vi "bode_ph.vi"() -> ()   [LabVIEW 2014]
doc: "Bode plot\nAcquisisce la risposta di un circuito utilizzando il generatore interno\nGenera il grafico della risposta in funzione della frequenza\nFM & ADL 09/2009, 10/2012, 10/2013 versione per 8.6 \nModifcato con set di DMA e Interrupts FM 10/2013\n9/2015 vers. LV2014"
uses:
  <vilib>/DAQmx/write.llb/DAQmx Write (Analog 1D DBL 1Chan NSamp).vi
  <vilib>/DAQmx/read.llb/DAQmx Read (Analog 1D Wfm NChan NSamp).vi
  <vilib>/DAQmx/create/channels.llb/DAQmx Create Channel (AO-Voltage-Basic).vi
  <vilib>/DAQmx/create/channels.llb/DAQmx Create Channel (AI-Voltage-Basic).vi
  <vilib>/DAQmx/configure/timing.llb/DAQmx Timing (Sample Clock).vi
  <vilib>/DAQmx/miscellaneous.llb/DAQmx Fill In Error Info.vi
  <vilib>/measure/matone.llb/Extract Single Tone Information 1 Chan.vi
  <vilib>/Utility/file.llb/Write To Spreadsheet File (DBL).vi
  <vilib>/measure/NI_MABase.lvlib
  <vilib>/measure/NI_MAPro.lvlib
  <resource>/objmgr/daqmx.rc
panel:
  in  "Fondo Scala":dbl(ring)=5.0 items=["10"=10.0, "5"=5.0, "0.5"=0.5, "0.05"=0.05]
  out "N. misura":i32=20
  in  "SALVA I DATI SU FILE":bool=TRUE caption="ON\nOFF"
  out "Fase":cluster{dbl[], dbl[]}(graph)={[5.0, 6.147467068473125, 7.558270271592312, 9.29284351784663, 11.42548989968722, 14.047564579899898, 17.271388129436826, 21.23505795050611, 26.10836388957094, 32.10006144457005, 39.46681412529165, 48.52418802655607, 59.66016958353027, 73.35178556285486, 90.18553723227052, 110.882524037588, 136.32933299805035, 167.61601701448424, 206.08278894903452, 253.37743168865742, 311.52588344006404, 383.0190218849582, 470.91936472731345, 578.9922573134888, 711.867166947118, 875.2359931869336, 1076.0968890518084, 1323.054037586474, 1626.6862251746509, 2000.0000000000045], [-2.511428467979215, -3.2956057199072006, -7.538567169946305, -10.113388336699302, -10.892831534570234, -13.380062579809533, -10.774958061787402, -13.590987224260658, -21.65618380795769, -25.567045102139673, -29.374990352035297, -30.80584091335669, -40.39456715017832, -46.922681187413104, -49.46128006672848, -55.656601427298085, -62.68913088564615, -64.84436978845952, -67.56276682724092, -74.50767078379593, -76.96614211460007, -77.43816453034884, -79.04548854172731, -83.2980148193289, -80.94888607866157, -84.03334246814163, -78.13471017673413, -78.78110200061434, -92.0554038069169, -84.81527118746277]}
  out "GAIN":cluster{dbl[], dbl[]}(graph)={[5.0, 6.147467068473125, 7.558270271592312, 9.29284351784663, 11.42548989968722, 14.047564579899898, 17.271388129436826, 21.23505795050611, 26.10836388957094, 32.10006144457005, 39.46681412529165, 48.52418802655607, 59.66016958353027, 73.35178556285486, 90.18553723227052, 110.882524037588, 136.32933299805035, 167.61601701448424, 206.08278894903452, 253.37743168865742, 311.52588344006404, 383.0190218849582, 470.91936472731345, 578.9922573134888, 711.867166947118, 875.2359931869336, 1076.0968890518084, 1323.054037586474, 1626.6862251746509, 2000.0000000000045], [0.997344434549249, 0.9962213082665805, 0.9941210435643523, 0.9922479926095603, 0.9878479615556824, 0.9824573247202957, 0.9738931698701306, 0.9613958789343343, 0.9430943055783031, 0.9186590086551807, 0.88260450854282, 0.8371109796491035, 0.7795638387175756, 0.7122020936433959, 0.6364315890190533, 0.5575733199071561, 0.48003430290297966, 0.4070800618335603, 0.3414788103570544, 0.28392605144903055, 0.23469423754251195, 0.19299749424063478, 0.15862845124464225, 0.1302776763618104, 0.10670713632692706, 0.08756567054703944, 0.07027549073207927, 0.057247542713008, 0.0468367874762694, 0.03824708830461569]}
  out "Vin (bianco) Vout (giallo)":waveform(dbl)[](graph)=[{"t0"=timestamp(3463116182.984375 s since 1904-01-01), "dt"=1.9999999999999998e-05, "Y"=[-0.40354768966159216, -0.3176421394330232, -0.2118748908641203, -0.09250948886795704, 0.032113552093432515, 0.1550167936225486, 0.26847628237502535, 0.3652222773509948, 0.43879623760444986, 0.4845894271489925, 0.5005894831758473, 0.4845894271489925, 0.43879623760444986, 0.3652222773509948, 0.26847628237502535, 0.15478961539836963, 0.03198373631517646, -0.09293138951490015, -0.21213452196228907, -0.31796667853872895, -0.40370995941588605, -0.4641067976603833, -0.49532754826133535, -0.4953600022764232, -0.4641067976603833, -0.4040669528769932, -0.31799913244936345, -0.21232924528602865, -0.09289893561902575, 0.031821466592759425, 0.15478961539836963, 0.268151740898926, 0.36509246025984043, 0.4383418762293826, 0.4846218816097759, 0.5003947562443536, 0.4846867905315109, 0.43860151129959596, 0.3649626431694226, 0.2683140116365024, 0.15482206943031035, 0.03172410475952403, -0.09302875120247918, -0.21216697584957225, -0.31803158636000955, -0.40374241336680144, -0.4640743436696399, -0.4953924562915376, -0.49532754826133535, -0.4641717056419421, -0.4039046831216613, -0.31803158636000955, -0.21229679139873198, -0.09293138951490015, 0.031886374481672516, 0.15462734523909027, 0.2682815574889114, 0.3648003718074358, 0.43853660253172927, 0.4846867905315109, 0.5002973927793823, 0.48471924499246266, 0.43853660253172927, 0.3649626431694226, 0.26834646578413124, 0.1546597992708896, 0.031756558703917935, -0.09280157393135828, -0.21203716030045566, -0.3178693168068953, -0.40374241336680144, -0.4640094356882249, -0.4951977322012501, -0.49532754826133535, -0.46394452770690575, -0.40370995941588605, -0.3180964941813367, -0.21223188362414672, -0.09302875120247918, 0.03185392053720702, 0.15452998314386185, 0.268216649193843, 0.3648977346244899, 0.4386339656836077, 0.4844920637669791, 0.5004596652212883, 0.4846867905315109, 0.4385690569156365, 0.3649626431694226, 0.26834646578413124, 0.15482206943031035, 0.03195128237065724, -0.09289893561902575, -0.2121020680750086, -0.31803158636000955, -0.4038722291706516, -0.4641067976603833, -0.4952301862162315, -0.4953924562915376, -0.4640094356882249, -0.4039695910237374, -0.3179342246281061, -0.2121020680750086, -0.09296384341076719, 0.031918828426155926, 0.15482206943031035, 0.268443828227245, 0.36518982307813713, 0.43866642006767165, 0.48471924499246266, 0.5004596652212883, 0.48471924499246266, 0.43869887445178785, 0.36518982307813713, 0.2682815574889114, 0.1548869774942766, 0.031886374481672516, -0.09280157393135828, -0.21203716030045566, -0.3178368628963073, -0.4038073212686888, -0.46391207371628207, -0.4953924562915376, -0.4951977322012501, -0.4641392516511507], "attributes"=variant("NI_ChannelName"=variant(string "Dev1/ai0"), "NI_UnitDescription"=variant(string "Volts"))}, {"t0"=timestamp(3463116182.984385 s since 1904-01-01), "dt"=1.9999999999999998e-05, "Y"=[-0.011212449060798765, -0.014522749144446944, -0.0166647079443697, -0.0177032334014217, -0.017670779481101948, -0.01627526089433491, -0.014003486395925527, -0.010530916672304998, -0.006246998656095383, -0.001800810747352719, 0.003067278528288692, 0.007902914220070749, 0.011992109777829095, 0.015562042618044544, 0.018255719347841527, 0.01994332410473799, 0.020332771362804047, 0.01971614653865677, 0.018060995724968443, 0.015140141453851102, 0.011343031100809003, 0.006961750199018043, 0.00222347636249437, -0.0026446128537431536, -0.007188162484401767, -0.011050179445062374, -0.01429557169241011, -0.01676206970656755, -0.01780059516229866, -0.017476055958895155, -0.016210353052468814, -0.013743855020318461, -0.010336193131576134, -0.006311906506719184, -0.0016060871828953507, 0.0029374628097945813, 0.007675736696527374, 0.011764932240134893, 0.015432226874918577, 0.01812590359919249, 0.020040685919026205, 0.020430133177701308, 0.019813508352590256, 0.01786627210269795, 0.015042779647125564, 0.01118076143256555, 0.006799480541560849, 0.0019638449289622025, -0.0026770667807093336, -0.007415339958356825, -0.01124490298390323, -0.014555203066110517, -0.016599800102835436, -0.017897956923052214, -0.017476055958895155, -0.01634016873614565, -0.01384121678627644, -0.010758094135836926, -0.00637681435728426, -0.0019630803839862975, 0.0033593638958058698, 0.007416105242000887, 0.01186229404190654, 0.015367319003454703, 0.018190811473483507, 0.01987841622863034, 0.02062485680795324, 0.019521422911245437, 0.017768910291788485, 0.01481560209867611, 0.011050945698261642, 0.006572303021783793, 0.0018664831416414804, -0.0029691521227308277, -0.007480247807926938, -0.011472080445235226, -0.014522749144446944, -0.0166647079443697, -0.017768141242020054, -0.0177032334014217, -0.016210353052468814, -0.014068394239686921, -0.010628278442476005, -0.006539083983440174, -0.002125350020243671, 0.002710285303025065, 0.007286289515117891, 0.011797386174042565, 0.015399772939178383, 0.018158357536329627, 0.019845962290601853, 0.020397679239385288, 0.019456515035576584, 0.017639094544143183, 0.014718240292444796, 0.010856222097290128, 0.006539849090450168, 0.0018015752835045273, -0.002871790342191765, -0.007350432108728361, -0.010952817675449186, -0.014522749144446944, -0.01676206970656755, -0.017897956923052214, -0.017962864763486065, -0.01653489226124592, -0.01423066384884499, -0.010952817675449186, -0.007025892859709993, -0.0022876196561251814, 0.002612923514641253, 0.00731874344681489, 0.01173247830624343, 0.015432226874918577, 0.01796363391375791, 0.01958633078698174, 0.020040685919026205, 0.01948896897340258, 0.017541732733584593, 0.014555970615721696, 0.010953583897703262, 0.006474941227830212, 0.0017366674254290385, -0.002871790342191765, -0.0073828860335498885], "attributes"=variant("NI_ChannelName"=variant(string "Dev1/ai1"), "NI_UnitDescription"=variant(string "Volts"))}]
  out "f_attuale":dbl=2000.0000000000045
  out "Ncamp/periodo":dbl=25.0
  in  "Nperiodi":dbl=5.0
  in  "Numero misure":i16=30
  in  "Freqmax":dbl=2000.0 min=0.0 max=100000.0
  in  "Freqmin":dbl=5.0 min=0.0 max=100000.0
  # "1) Scegliere la frequenza iniziale e finale (<8 kHz) e il numero di misure.\n2) Scegliere quanti periodi della sinusoide si prendono e quanti campioni si generano per ogni periodo; per le frequenze alte ridurre il NCamp/periodo: il prodotto Freqmax * Ncamp non deve superare  ~ 60000.\n3) Premere la freccia bianca di avvio."
  # "Foma d'onda generata Vin(t)"
  # "NO\nSI"
  # "Fase"
  # "I Collegamenti"
  # "Collegare il CB 22 (Analog Output 0) all'ingresso. \nI due canali di misura (riferiti a terra) sono il CB68 (Vin) e CB33 (Vout).\nLa terra del circuito DEVE essere in comune alla terra della scheda (CB29)."
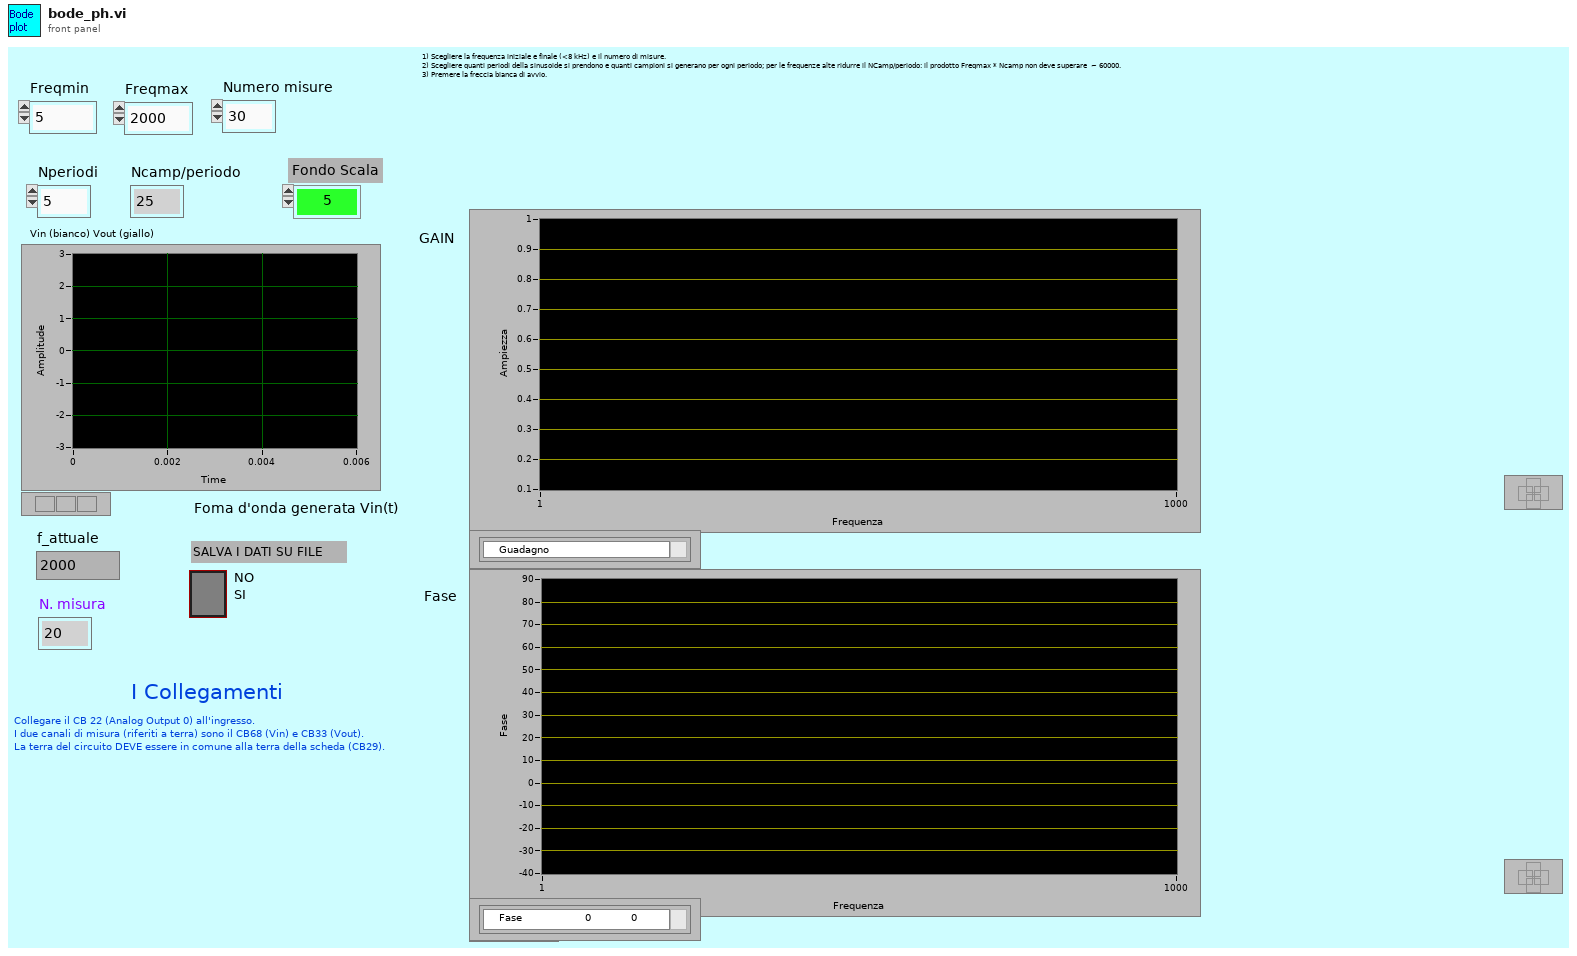
[diagram p1: front panel]
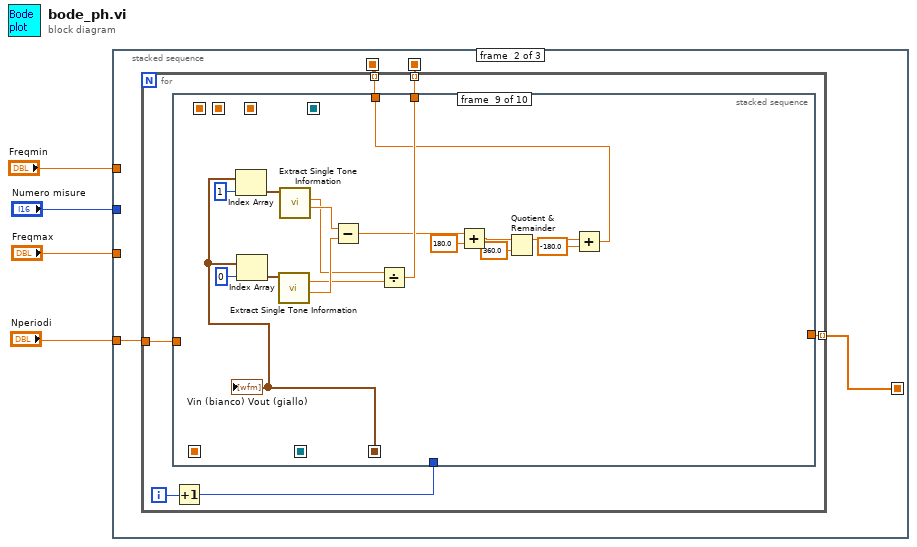
[diagram p0: block diagram]
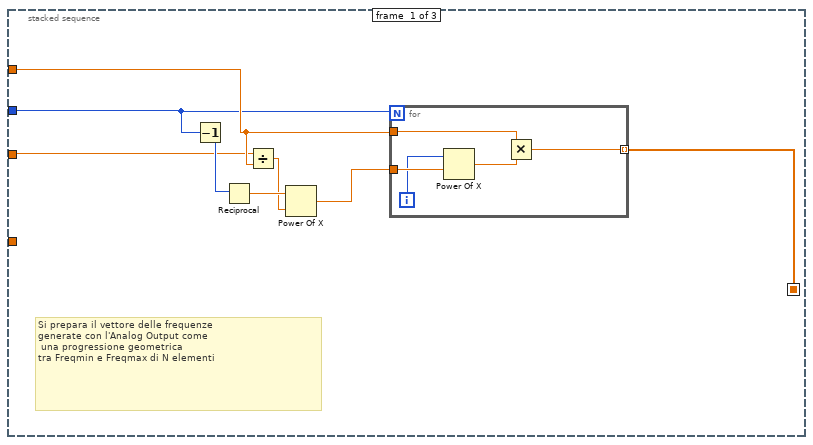
[diagram p2: hidden frame]
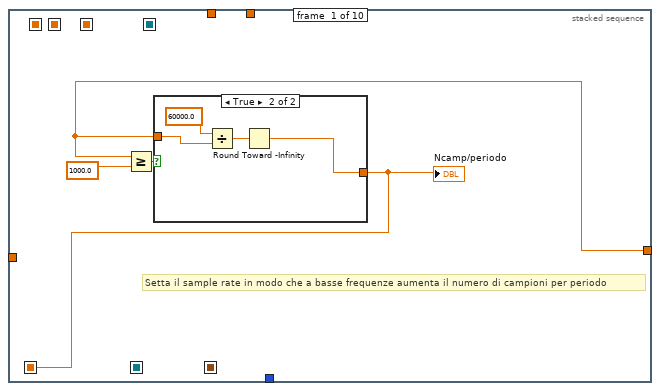
[diagram p3: hidden frame]
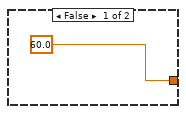
[diagram p4: hidden frame]
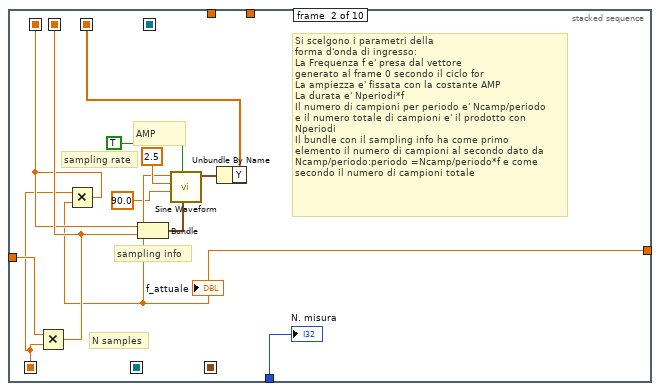
[diagram p5: hidden frame]
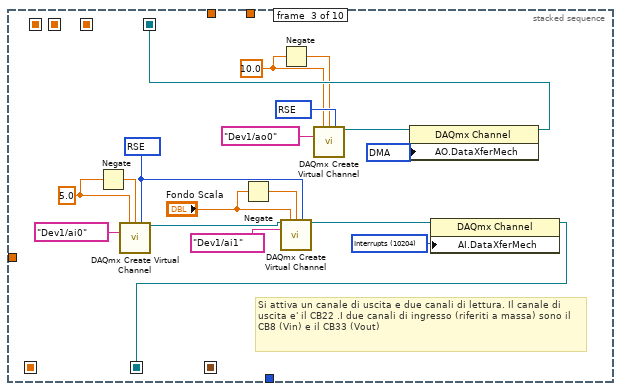
[diagram p6: hidden frame]
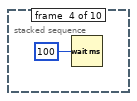
[diagram p7: hidden frame]
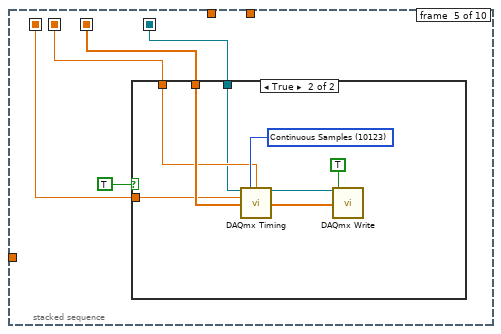
[diagram p8: hidden frame]
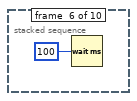
[diagram p10: hidden frame]
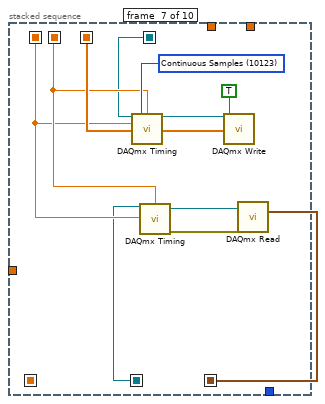
[diagram p11: hidden frame]
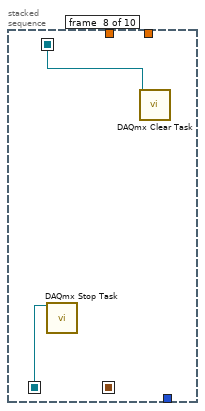
[diagram p12: hidden frame]
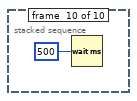
[diagram p13: hidden frame]
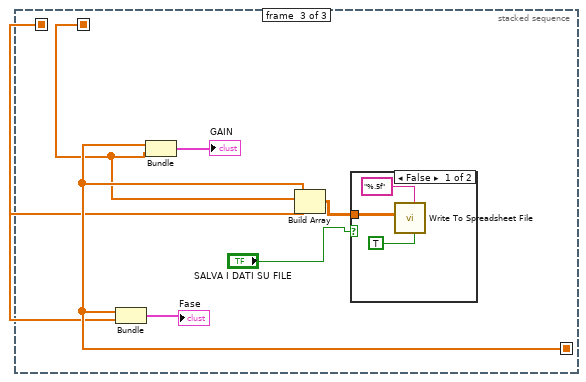
[diagram p14: hidden frame]
diagram:
  n1 = stacked-sequence {
    seq-local: [w5 _ _] -> [_ w21 w116]
    seq-local: [_ w19 _] -> [_ _ w115]
    seq-local: [_ w18 _] -> [_ _ w114]
    tunnel: "Freqmin" -> [w8 _ _]
    tunnel: "Numero misure" -> [w7 _ _]
    tunnel: "Freqmax" -> [w6 _ _]
    tunnel: "Nperiodi" -> [_ w20 _]
    frame #0 {
      # "Si prepara il vettore delle frequenze\ngenerate con l'Analog Output come\n una progressione geometrica\ntra Freqmin e Freqmax di N elementi"
      n2 = Decrement(x=w7) -> (x-1=w12:i16)
      n3 = Reciprocal(x=w12) -> (1/x=w11:dbl)
      n4 = Divide(x=w6, y=w8) -> (x/y=w10:dbl)
      n5 = Power Of X(1:w10, 2:w11) -> (0:w9:dbl)
      n6 = for {
        N: w7 -> [_]
        tunnel: w9 -> [w17]
        tunnel: w8 -> [w15]
        tunnel: [w13] -> w5 mode=indexing
        i -> [w16]
        n7 = Power Of X(1:w17, 2:w16) -> (0:w14:dbl)
        n8 = Multiply(x=w15, y=w14) -> (x*y=w13:dbl)
      }
    }
    frame #1 {
      n9 = for {
        tunnel: w21 -> [w24] mode=indexing
        tunnel: w20 -> [w27]
        tunnel: [w26] -> w19 mode=indexing
        tunnel: [w25] -> w18 mode=indexing
        i -> [w23]
        n10 = Increment(x=w23) -> (x+1=w22:i32)
        n11 = stacked-sequence {
          seq-local: [_ w46 _ _ _ _ _ _ _ _] -> [_ _ _ _ w72 _ w86 _ _ _]
          seq-local: [_ w43 _ _ _ _ _ _ _ _] -> [_ _ _ _ w71 _ w84 _ _ _]
          seq-local: [_ w42 _ _ _ _ _ _ _ _] -> [_ _ _ _ w70 _ w83 _ _ _]
          seq-local: [_ _ _ _ _ _ w87 _ _ _] -> [_ _ _ _ _ _ _ _ w108 _]
          seq-local: [w28 _ _ _ _ _ _ _ _ _] -> [_ w38 _ _ _ _ _ _ _ _]
          seq-local: [_ _ w61 _ _ _ _ _ _ _] -> [_ _ _ _ w69 _ w82 w92 _ _]
          seq-local: [_ _ w59 _ _ _ _ _ _ _] -> [_ _ _ _ _ _ w81 w93 _ _]
          tunnel: w24 -> [w29 w41 _ _ _ _ _ _ _ _]
          tunnel: w27 -> [_ w44 _ _ _ _ _ _ _ _]
          tunnel: [_ _ _ _ _ _ _ _ w104 _] -> w26
          tunnel: [_ _ _ _ _ _ _ _ w94 _] -> w25
          tunnel: w22 -> [_ w37 _ _ _ _ _ _ _ _]
          frame #0 {
            # "Setta il sample rate in modo che a basse frequenze aumenta il numero di campioni per periodo"
            n12 = Greater Or Equal?(x=w29, y=1000.0) -> (x >= y?=w30:bool)
            n13 = case shown="True" w30 {
              tunnel: [60.0 w33] -> w28
              tunnel: w29 -> [_ w36]
              frame False {
              }
              frame True {
                n14 = Divide(x=60000.0, y=w36) -> (x/y=w34:dbl)
                n15 = Round Toward -Infinity(1:w34) -> (0:w33:dbl)
              }
            }
            "Ncamp/periodo" <- w28
          }
          frame #1 {
            # "Si scelgono i parametri della\nforma d'onda di ingresso:\nLa Frequenza f e' presa dal vettore \ngenerato al frame 0 secondo il ciclo for\nLa ampiezza e' fissata con la costante AMP\nLa durata e' Nperiodi*f\nIl numero di campioni per periodo e' Ncamp/periodo\ne il numero totale di campioni e' il prodotto con \nNperiodi\nIl bundle con il sampling info ha come primo\nelemento il numero di campioni al secondo dato da \nNcamp/periodo:periodo =Ncamp/periodo*f e come\nsecondo il numero di campioni totale"
            # "sampling rate"
            # "N samples"
            # "AMP"
            # "sampling info"
            n16 = Multiply(x=w44, y=w38) -> (x*y=w43:dbl)
            n17 = Multiply(x=w38, y=w41) -> (x*y=w42:dbl)
            n18 = Bundle(w42, w43) -> (w45:cluster{dbl, dbl})  [unwired: 1 out]
            n19 = call <vilib>:"Sine Waveform.vi"("sampling info"=w45, "reset signal"=TRUE, "phase"=90.0, "amplitude"=2.5, "frequency"=w41) -> ("signal out"=w47:waveform(dbl))  [unwired: 2 in, 4 out]
            n20 = Unbundle By Name(w47) -> ("Y"=w46:dbl[])
            "f_attuale" <- w41
            "N. misura" <- w37
          }
          frame #2 {
            w60 = 10204 items=["DMA"=10054, "Interrupts"=10204, "Programmed I/O"=10264, "USB Bulk"=12590] ("AO.DataXferMech")
            w63 = 10054 items=["DMA"=10054, "Interrupts"=10204, "Programmed I/O"=10264, "USB Bulk"=12590] ("AO.DataXferMech")
            w58 = 5.0 ("maximum value")
            w52 = 10083 items=["default"=-1, "RSE"=10083, "NRSE"=10078, "Differential"=10106, "Pseudodifferential"=12529] ("input terminal configuration")
            w56 = 10.0 ("maximum value")
            w65 = 10083 items=["Default"=-1, "RSE"=10083, "Differential"=10106, "Pseudodifferential"=12529] ("output terminal configuration")
            # "Si attiva un canale di uscita e due canali di lettura. Il canale di uscita e' il CB22 .I due canali di ingresso (riferiti a massa) sono il CB8 (Vin) e il CB33 (Vout)"
            n21 = Negate(x=w58) -> (-x=w57:dbl)
            n22 = call-poly <vilib>:"DAQmx Create Virtual Channel.vi"("maximum value"=w58, "minimum value"=w57, "input terminal configuration"=w52, "physical channels"=tag "Dev1/ai0") -> ("task out"=w53:refnum<k21>)  [unwired: 5 in, 6 out]
            n23 = Negate(x="Fondo Scala") -> (-x=w51:dbl)
            n24 = Negate(x=w56) -> (-x=w55:dbl)
            n25 = call-poly <vilib>:"DAQmx Create Virtual Channel.vi"("task in"=w53, "maximum value"="Fondo Scala", "minimum value"=w51, "input terminal configuration"=w52, "physical channels"=tag "Dev1/ai1") -> ("task out"=w49:refnum<k21>)  [unwired: 4 in, 6 out]
            n26 = call-poly <vilib>:"DAQmx Create Virtual Channel.vi"("maximum value"=w56, "minimum value"=w55, "output terminal configuration"=w65, "physical channels"=tag "Dev1/ao0") -> ("task out"=w62:refnum<k21>)  [unwired: 5 in, 6 out]
            n27 = property class="DAQmx Channel"(reference=w62, "AO.DataXferMech"=w63) -> (reference out=w61:refnum<k21>)  [unwired: 1 in, 1 out]
            n28 = property class="DAQmx Channel"(reference=w49, "AI.DataXferMech"=w60) -> (reference out=w59:refnum<k21>)  [unwired: 1 in, 1 out]
          }
          frame #3 {
            n29 = Wait (ms)(milliseconds to wait=u32 100 ("millisecond multiple")) -> ()  [unwired: 1 out]
          }
          frame #4 {
            n30 = case shown="True" TRUE {
              tunnel: w72 -> [_ w77]
              tunnel: w71 -> [_ w75]
              tunnel: w70 -> [_ w74]
              tunnel: w69 -> [_ w73]
              frame False {
              }
              frame True {
                w76 = 10123 items=["Finite Samples"=10178, "Continuous Samples"=10123, "Hardware Timed Single Point"=12522] ("sample mode")
                n31 = call-poly <vilib>:"DAQmx Timing.vi"("task/channels in"=w73, "sample mode"=w76, "samples per channel"=w75, "rate"=w74) -> ("task out"=w78:refnum<k21>)  [unwired: 3 in, 8 out]
                n32 = call-poly <vilib>:"DAQmx Write.vi"("task/channels in"=w78, "auto start"=TRUE, "data"=w77) -> ()  [unwired: 1 in, 12 out]
              }
            }
          }
          frame #5 {
            n33 = Wait (ms)(milliseconds to wait=u32 100 ("millisecond multiple")) -> ()  [unwired: 1 out]
          }
          frame #6 {
            w85 = 10123 items=["Finite Samples"=10178, "Continuous Samples"=10123, "Hardware Timed Single Point"=12522] ("sample mode")
            n34 = call-poly <vilib>:"DAQmx Timing.vi"("task/channels in"=w82, "sample mode"=w85, "samples per channel"=w84, "rate"=w83) -> ("task out"=w88:refnum<k21>)  [unwired: 3 in, 8 out]
            n35 = call-poly <vilib>:"DAQmx Timing.vi"("task/channels in"=w81, "samples per channel"=w84, "rate"=w83) -> ("task out"=w91:refnum<k21>, "error out"=w90:errorcluster)  [unwired: 4 in, 7 out]
            n36 = call-poly <vilib>:"DAQmx Write.vi"("task/channels in"=w88, "auto start"=TRUE, "data"=w86) -> ()  [unwired: 1 in, 12 out]
            n37 = call-poly <vilib>:"DAQmx Read.vi"("task/channels in"=w91, "error in"=w90) -> ("data"=w87:waveform(dbl)[])  [unwired: 1 in, 12 out]
          }
          frame #7 {
            n38 = call <vilib>:"DAQmx Stop Task.vi"("task/channels in"=w93) -> ()  [unwired: 1 in, 14 out]
            n39 = call <vilib>:"DAQmx Clear Task.vi"("task in"=w92) -> ()  [unwired: 1 in, 14 out]
          }
          frame #8 {
            n40 = Index Array(array=w108, index=1) -> (element=w109:waveform(dbl))
            n41 = Index Array(array=w108, index=0) -> (element=w110:waveform(dbl))
            n42 = call-poly <vilib>:"Extract Single Tone Information.vi"("time signal in"=w110) -> ("detected phase (deg)"=w105:dbl, "detected amplitude"=w101:dbl)  [unwired: 3 in, 6 out]
            n43 = call-poly <vilib>:"Extract Single Tone Information.vi"("time signal in"=w109) -> ("detected phase (deg)"=w106:dbl, "detected amplitude"=w102:dbl)  [unwired: 3 in, 6 out]
            n44 = Subtract(x=w106, y=w105) -> (x-y=w95:dbl)
            n45 = Divide(x=w102, y=w101) -> (x/y=w104:dbl)
            n46 = Add(x=w95, y=180.0) -> (x+y=w97:dbl)
            n47 = Quotient & Remainder(x=w97, y=360.0) -> (x-y*floor(x/y)=w99:dbl)  [unwired: 1 out]
            n48 = Add(x=w99, y=-180.0) -> (x+y=w94:dbl)
            "Vin (bianco) Vout (giallo)" <- w108
          }
          frame #9 {
            n49 = Wait (ms)(milliseconds to wait=u32 500 ("millisecond multiple")) -> ()  [unwired: 1 out]
          }
        }
      }
    }
    frame #2 {
      n50 = Bundle(w116, w114) -> (→"Fase":cluster{dbl[], dbl[]})  [unwired: 1 out]
      n51 = Bundle(w116, w115) -> (→"GAIN":cluster{dbl[], dbl[]})  [unwired: 1 out]
      n52 = Build Array(w116, w115, w114) -> (w113:dbl[][])
      n53 = case shown="False" "SALVA I DATI SU FILE" {
        tunnel: w113 -> [w121 _]
        frame False {
          n54 = call-poly <vilib>:"Write To Spreadsheet File.vi"("transpose? (no:F)"=TRUE, "format (%.3f)"="%.5f", "2D data"=w121) -> ()  [unwired: 3 in, 3 out]
        }
        frame True {
        }
      }
    }
  }
